vi "-Parse_Authentication_Response.vi"(8 "error in (no error)":errorcluster, 11 "Postgres Connector In":refnum<class "Postgres Connector.lvclass">) -> (0 "error out":errorcluster, 3 "Postgres Connector Out":refnum<class "Postgres Connector.lvclass">)   [LabVIEW 2020, in "Postgres Connector.lvclass"]
doc: "This VI is used to filter the response of the database. Depending of the type of authentication recquired, the good case will be choosen and therefore the good method of authentication."
uses:
  Postgres Connector.lvclass
  Postgres Connector.lvclass/Postgres Connector.ctl
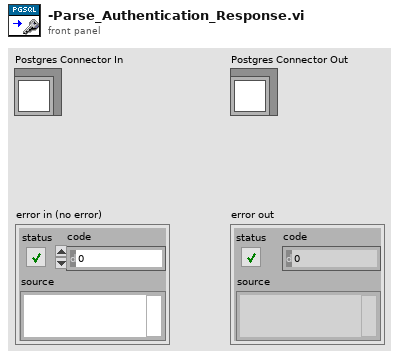
[diagram p1: front panel]
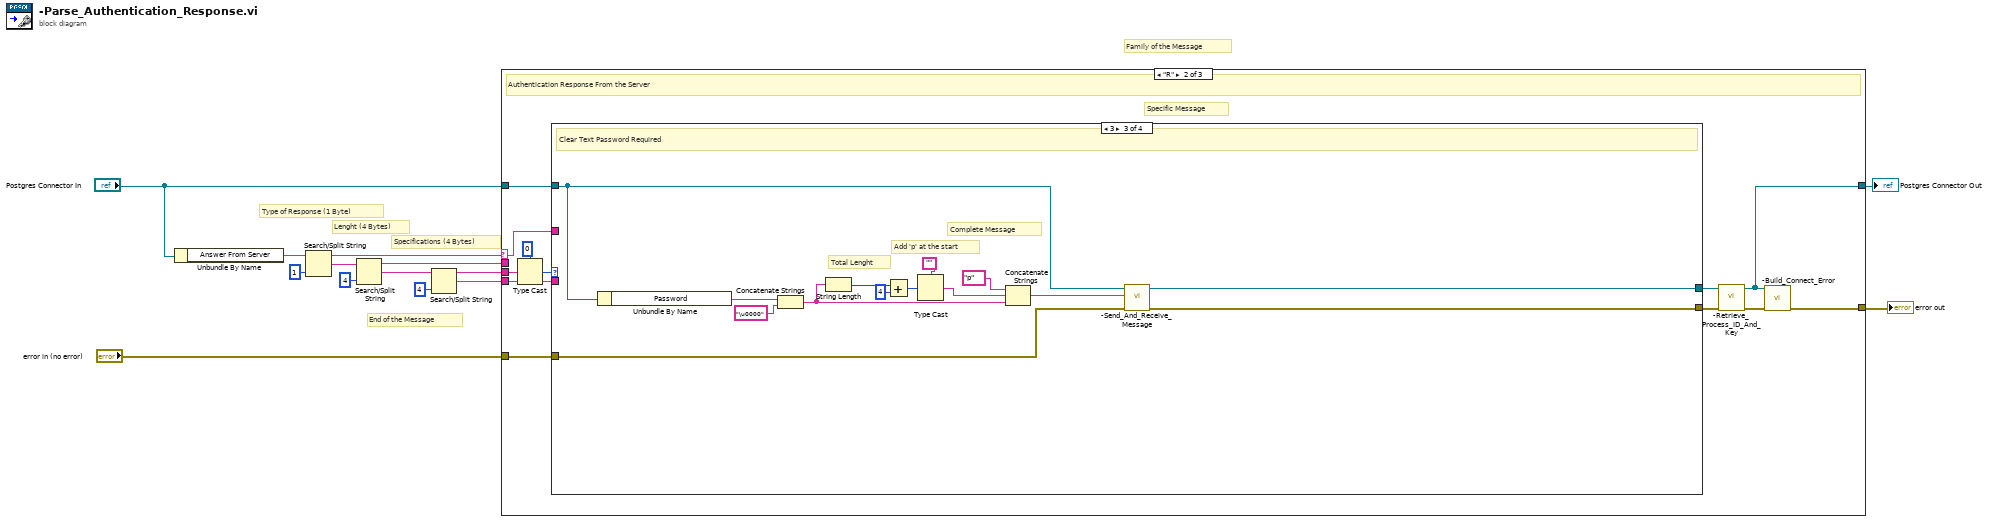
[diagram p0: block diagram]
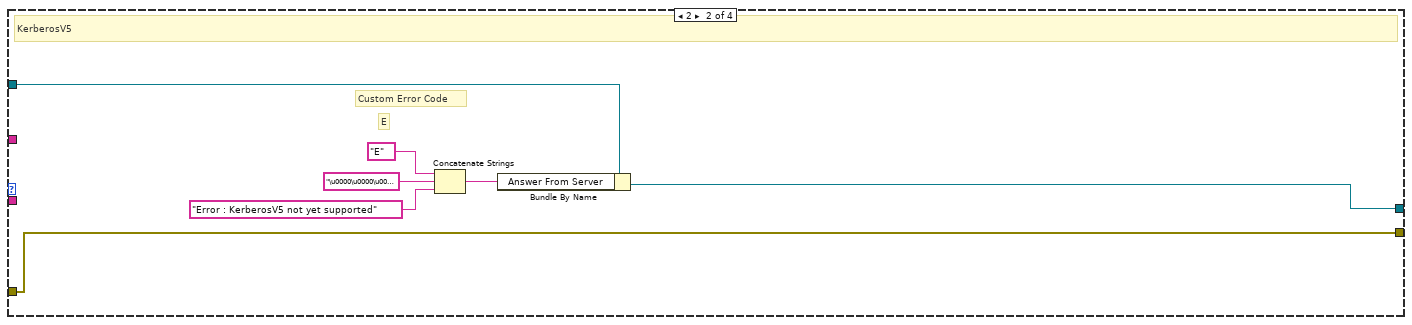
[diagram p4: hidden frame]
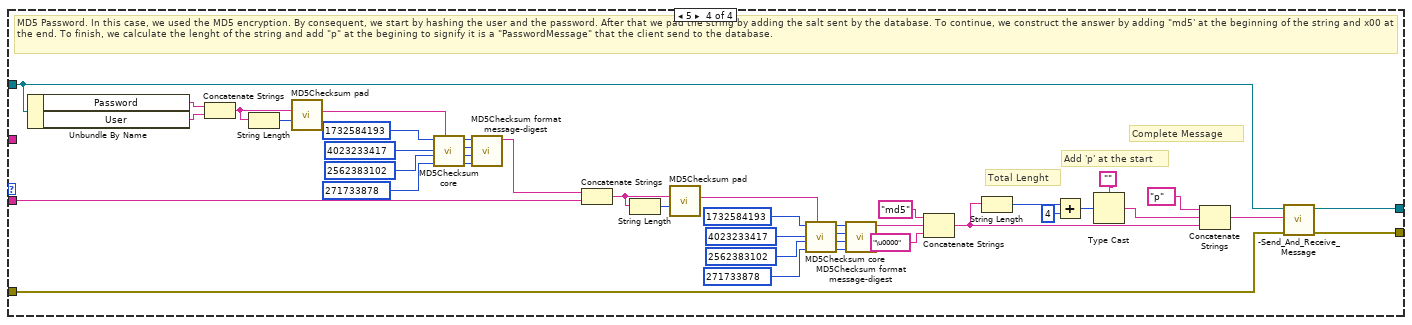
[diagram p5: hidden frame]
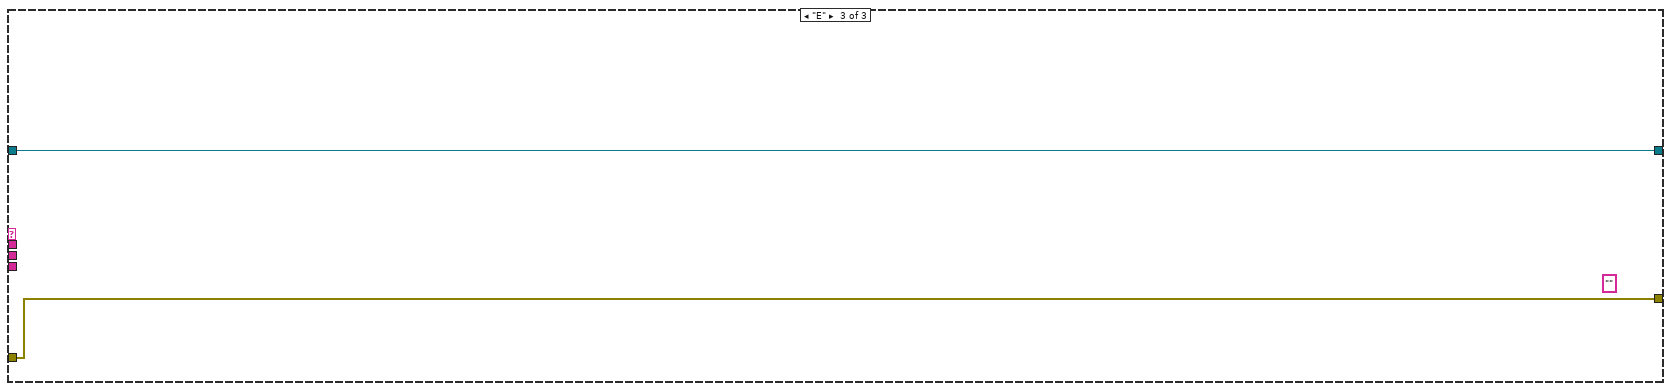
[diagram p6: hidden frame]
diagram:
  # "Family of the Message"
  # "End of the Message"
  # "Specifications (4 Bytes)"
  # "Lenght (4 Bytes)"
  # "Type of Response (1 Byte)"
  n1 = Unbundle By Name("Postgres Connector In") -> ("Answer From Server"=w2:string)
  n2 = Search/Split String(string=w2, offset (0)=1 ("length (rest)")) -> (substring before match=w11:string, match + rest of string=w10:string)  [unwired: 1 in, 1 out]
  n3 = Search/Split String(string=w10, offset (0)=4 ("length (rest)")) -> (substring before match=w6:string, match + rest of string=w9:string)  [unwired: 1 in, 1 out]
  n4 = Search/Split String(string=w9, offset (0)=4 ("length (rest)")) -> (substring before match=w8:string, match + rest of string=w7:string)  [unwired: 1 in, 1 out]
  n5 = case shown="\"R\"" w11 {
    selector: w11 -> [_ w22 _]
    tunnel: w8 -> [_ w28 _]
    tunnel: w7 -> [_ w25 _]
    tunnel: w6 -> [_ _ _]
    tunnel: "Postgres Connector In" -> [w15 w24 w93]
    tunnel: [w16 w21 w94] -> w5
    tunnel: "error in (no error)" -> [w16 w23 w94]
    tunnel: [w15 w17 w93] -> w1
    frame "0", Default {
    }
    frame "R" {
      # "Specific Message"
      # "Authentication Response From the Server"
      n6 = Type Cast(type=0, x=w28) -> (*(type *) &x=w26:i32)
      n7 = case shown="3" w26 {
        tunnel: w25 -> [_ _ _ w60]
        tunnel: w24 -> [w29 w36 w40 w58]
        tunnel: [w30 w37 w38 w55] -> w20
        tunnel: w23 -> [w30 w37 w42 w57]
        tunnel: w22 -> [_ _ _ _]
        tunnel: [w29 w34 w39 w56] -> w19
        frame 0, Default {
          # "Authentication OK"
        }
        frame 2 {
          # "Custom Error Code"
          # "E"
          # "KerberosV5"
          n8 = Concatenate Strings("E" ("Answer From Server"), "\u0000\u0000\u0000\u0000" ("Answer From Server"), "Error : KerberosV5 not yet supported" ("string")) -> (w33:string)
          n9 = Bundle By Name(cluster=w36, "Answer From Server"=w33) -> (w34:refnum<class "Postgres Connector.lvclass">)
        }
        frame 3 {
          # "Complete Message"
          # "Total Lenght"
          # "Add 'p' at the start"
          # "Clear Text Password Required"
          n10 = Unbundle By Name(w40) -> ("Password"=w43:string)
          n11 = Concatenate Strings(w43, "\u0000" ("string")) -> (w45:string)
          n12 = String Length(string=w45) -> (length=w50:i32)
          n13 = Add(x=w50, y=4) -> (x+y=w48:i32)
          n14 = Type Cast(type="", x=w48) -> (*(type *) &x=w51:string)
          n15 = Concatenate Strings("p", w51, w45) -> (w41:string)
          n16 = call "-Send_And_Receive_Message.vi"("error in (no error)"=w42, "Message To Send"=w41, "Postgres Connector In"=w40) -> ("error out"=w38:errorcluster, "Postgres Connector Out"=w39:refnum<class "Postgres Connector.lvclass">)  [unwired: 7 in]
        }
        frame 5 {
          # "Complete Message"
          # "Total Lenght"
          # "Add 'p' at the start"
          # "MD5 Password. In this case, we used the MD5 encryption. By consequent, we start by hashing the user and the password. After that we pad the string by adding the salt sent by the database. To continue, we construct the answer by adding \"md5' at the beginning of the string and x00 at the end. To finish, we calculate the lenght of the string and add \"p\" at the begining to signify it is a \"PasswordMessage\" that the client send to the database."
          n17 = Unbundle By Name(w58) -> ("Password"=w52:string, "User"=w53:string)
          n18 = Concatenate Strings(w52, w53) -> (w77:string)
          n19 = String Length(string=w77) -> (length=w76:i32)
          n20 = call <vilib>:"MD5Checksum pad.vi"("Message String Length (bytes)"=w76, "Last Part of Message String"=w77) -> ("Padding"=w78:string)  [unwired: 9 in]
          n21 = call <vilib>:"MD5Checksum core.vi"("Input String"=w78, "s4 in"=u32 271733878 ("s4"), "s3 in"=u32 2562383102 ("s3"), "s2 in"=u32 4023233417 ("s2"), "s1 in"=u32 1732584193 ("s1")) -> ("s4 out"=w89:u32, "s3 out"=w90:u32, "s2 out"=w91:u32, "s1 out"=w92:u32)  [unwired: 3 in]
          n22 = call <vilib>:"MD5Checksum format message-digest.vi"("s4"=w89, "s3"=w90, "s2"=w91, "s1"=w92) -> ("MD5 message-digest"=w64:string)  [unwired: 7 in]
          n23 = Concatenate Strings(w64, w60) -> (w65:string)
          n24 = String Length(string=w65) -> (length=w75:i32)
          n25 = call <vilib>:"MD5Checksum pad.vi"("Message String Length (bytes)"=w75, "Last Part of Message String"=w65) -> ("Padding"=w74:string)  [unwired: 9 in]
          n26 = call <vilib>:"MD5Checksum core.vi"("Input String"=w74, "s4 in"=u32 271733878 ("s4"), "s3 in"=u32 2562383102 ("s3"), "s2 in"=u32 4023233417 ("s2"), "s1 in"=u32 1732584193 ("s1")) -> ("s4 out"=w69:u32, "s3 out"=w68:u32, "s2 out"=w67:u32, "s1 out"=w66:u32)  [unwired: 3 in]
          n27 = call <vilib>:"MD5Checksum format message-digest.vi"("s4"=w69, "s3"=w68, "s2"=w67, "s1"=w66) -> ("MD5 message-digest"=w63:string)  [unwired: 7 in]
          n28 = Concatenate Strings("md5" ("string"), w63, "\u0000" ("string")) -> (w62:string)
          n29 = String Length(string=w62) -> (length=w83:i32)
          n30 = Add(x=w83, y=4) -> (x+y=w81:i32)
          n31 = Type Cast(type="", x=w81) -> (*(type *) &x=w84:string)
          n32 = Concatenate Strings("p", w84, w62) -> (w59:string)
          n33 = call "-Send_And_Receive_Message.vi"("error in (no error)"=w57, "Message To Send"=w59, "Postgres Connector In"=w58) -> ("error out"=w55:errorcluster, "Postgres Connector Out"=w56:refnum<class "Postgres Connector.lvclass">)  [unwired: 7 in]
        }
      }
      n34 = call "-Retrieve_Process_ID_And_Key.vi"("error in (no error)"=w20, "Postgres Connector In"=w19) -> ("error out"=w18:errorcluster, "Postgres Connector Out"=w17:refnum<class "Postgres Connector.lvclass">)  [unwired: 8 in]
      n35 = call "-Build_Connect_Error.vi"("error in (no error)"=w18, "Postgres Connector In"=w17) -> ("error out"=w21:errorcluster)  [unwired: 9 in]
    }
    frame "E" {
      (unwired) "" ("Answer From Server")
    }
  }
  "error out" <- w5
  "Postgres Connector Out" <- w1
